vi "1_SimpleDemo_MHHisto.vi"() -> ()   [LabVIEW 2017]
uses:
  _lib/PQ/MultiHarp/MH_RefSource.ctl
  _lib/PQ/MultiHarp/MH_MeasMode.ctl
  _lib/PQ/MultiHarp/mhlib_x86_x64_UIThread.llb/MH_DllPath_global.vi
  <vilib>/Utility/error.llb/Error Cluster From Error Code.vi
  _lib/PQ/MultiHarp/MH_LibVersion_global.vi
  <vilib>/ErrorRing/Error Ring.xnode
panel:
  in  "Binning":i32(ring) caption="Resolution [ps]" items=["80", "160", "320", "640", "1280", "2560", "5120", "10240", "20480", "40960", "81920", "163840", "327680", "655360", "1310720", "2621440", "5242880", "10485760", "20971520", "41943040", "83886080", "167772160", "335544320"]
  in  "HistoLength":i32(ring)=6 caption="Histo Length" items=["1024", "2048", "4096", "8192", "16384", "32768", "65536"]
  in  "Acqu.Time":i32=10000 caption="Acqu.Time [ms]" min=1 max=360000 step=1
  in  "GlobalOffset":i32 caption="GlobalOffset [ns]" min=0 max=100000000 step=1
  in  "OverflowLevel":u32=65535 min=1 step=1
  in  "StopOnOverflow":bool=TRUE
  in  "Trg.Edge":i32(ring) items=["falling", "rising"]
  in  "Trg.Level":i32=-50 caption="Trg.Level [mV]" min=-1200 max=1200 step=1
  in  "Offset":i32 caption="Offset [ps]" min=-99999 max=99999 step=1
  in  "Enable":bool=TRUE
  in  "SyncTrg.Edge":i32(ring) items=["falling", "rising"]
  in  "SyncTrg.Level":i32=-50 caption="SyncTrg.Level [mV]" min=-1200 max=1200 step=1
  in  "SyncOffset":i32 caption="SyncOffset [ps]" min=-99999 max=99999 step=1
  in  "SyncDivider":i32(ring)=8 items=["1"=1, "2"=2, "4"=4, "8"=8, "16"=16]
  out "HistoGraph":T1(graph)={0.0, "Resolution"=0.08, "Histogram"=[]}
  out "CountRates":i32[](array[numeric]) caption="Count Rates [cps]"
  out "SyncRate":i32 caption="Sync Rate [cps]"
  in  "stop":bool
  out "error out":errorcluster
  # "Acquisition"
  # "All Channels"
  # "Sync"
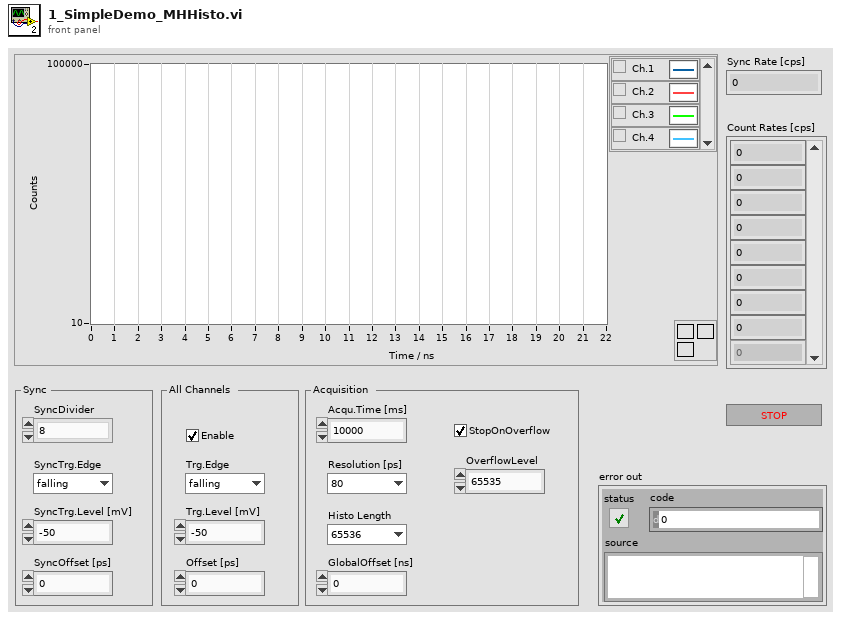
[diagram p1: front panel]
types:
  T1 = cluster{dbl, "Resolution":dbl, "Histogram":u32[][]}
  T2 = typedef "MH_MeasMode.ctl" = i32
  T3 = typedef "MH_RefSource.ctl" = enum16{"INTERNAL", "EXTERNAL_10MHZ", "WR_MASTER_GENERIC", "WR_SLAVE_GENERIC", "WR_GRANDM_GENERIC", "EXTN_GPS_PPS", "EXTN_GPS_PPS_UART", "WR_MASTER_MHARP", "WR_SLAVE_MHARP", "WR_GRANDM_MHARP"}
  T4 = typedef "MH_InitInfo.ctl" = cluster{"Library Version":string, "Serial No.":string, "Model":string, "Partnum":string, "Version":string, "features":i32, "nchannels":i32, "Base Resolution":dbl, "Bin Steps":i32}
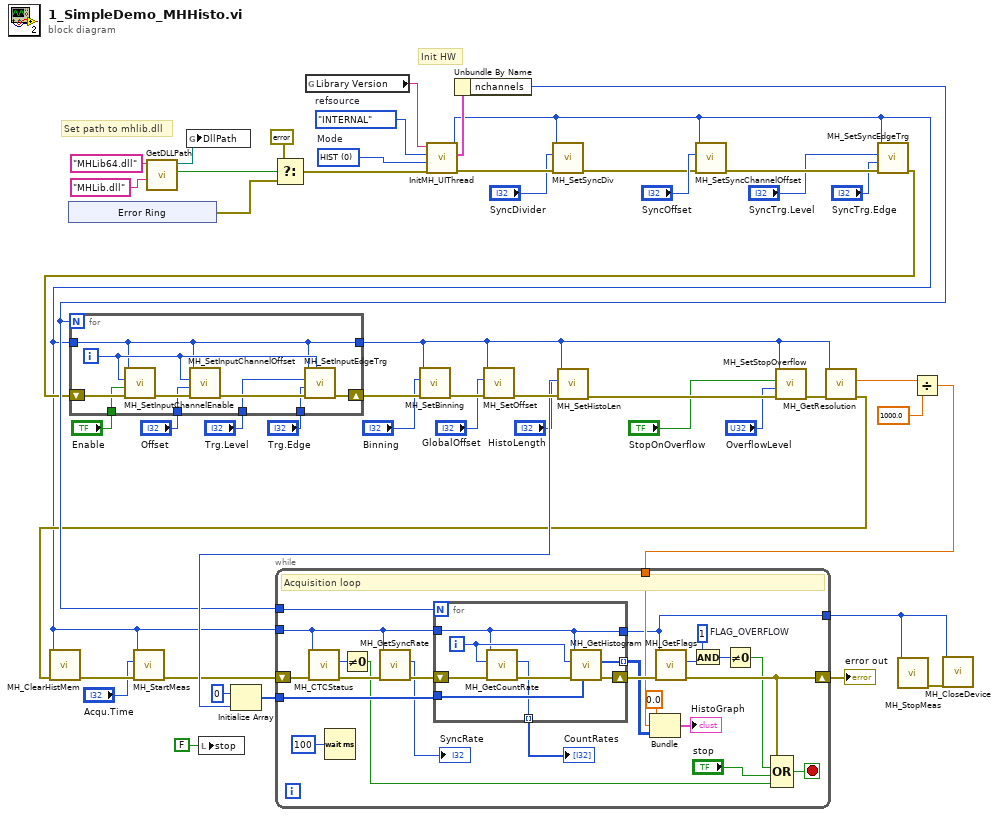
[diagram p0: block diagram]
diagram:
  w1 = T2 0 items=["HIST"=0, "T2"=2, "T3"=3]  # Mode
  w50 = MH_RefSource."INTERNAL"  # refsource
  # "Init HW"
  # "Set path to mhlib.dll"
  n1 = xnode "Error Ring"() -> ("error out"=w49:errorcluster)
  n2 = call "GetDLLPath.vi"("DllName_32bit"="MHLib.dll" ("name or relative path"), "DllName_64bit"="MHLib64.dll" ("name or relative path")) -> ("file exists?"=w47:bool, "DLLPath"=w46:path)  [unwired: 8 in]
  n3 = global write "MH_DllPath_global.vi" "DllPath"(w46) -> ()
  n4 = local write "stop"(FALSE ("stop")) -> ()
  n5 = Select(t=errorcluster {"status"=FALSE, "code"=0, "source"=""} ("error IO"), s=w47, f=w49) -> (s? t:f=w43:errorcluster)
  n6 = global read "MH_LibVersion_global.vi" "Library Version"() -> (w4:string)
  n7 = call "InitMH_UIThread.vi"("error in (no error)"=w43, "Mode"=w1, "refsource"=w50, "Library Version"=w4) -> ("error out"=w37:errorcluster, "Init Info"=w39:T4, "DevIdx"=w10:i32)  [unwired: 5 in]
  n8 = Unbundle By Name(w39) -> ("nchannels"=w19:i32)
  n9 = call "MH_SetSyncDiv.vi"("error in (no error)"=w37, "SyncDivider"="SyncDivider", "devidx"=w10) -> ("error out"=w36:errorcluster)  [unwired: 7 in, 1 out]
  n10 = call "MH_SetSyncChannelOffset.vi"("error in (no error)"=w36, "Offset"="SyncOffset", "devidx"=w10) -> ("error out"=w41:errorcluster)  [unwired: 7 in, 1 out]
  n11 = call "MH_SetSyncEdgeTrg.vi"("error in (no error)"=w41, "edge"="SyncTrg.Edge", "level"="SyncTrg.Level", "devidx"=w10) -> ("error out"=w18:errorcluster)  [unwired: 6 in, 1 out]
  n12 = for {
    N: w19 -> [_]
    shift-right: [w57] -> w38
    shift-left: w18 -> [w60]
    tunnel: w10 -> [w55]
    tunnel: [w55] -> w13
    tunnel: "Enable" -> [w54]
    tunnel: "Offset" -> [w53]
    tunnel: "Trg.Edge" -> [w52]
    tunnel: "Trg.Level" -> [w51]
    i -> [w56]
    n13 = call "MH_SetInputChannelEnable.vi"("error in (no error)"=w60, "enable"=w54, "channel"=w56, "devidx"=w55) -> ("error out"=w59:errorcluster)  [unwired: 6 in, 1 out]
    n14 = call "MH_SetInputChannelOffset.vi"("error in (no error)"=w59, "Offset"=w53, "channel"=w56, "devidx"=w55) -> ("error out"=w58:errorcluster)  [unwired: 6 in, 1 out]
    n15 = call "MH_SetInputEdgeTrg.vi"("channel"=w56, "error in (no error)"=w58, "edge"=w52, "level"=w51, "devidx"=w55) -> ("error out"=w57:errorcluster)  [unwired: 5 in, 1 out]
  }
  n16 = call "MH_SetBinning.vi"("error in (no error)"=w38, "Binning"="Binning", "devidx"=w13) -> ("error out"=w34:errorcluster)  [unwired: 7 in, 1 out]
  n17 = call "MH_SetOffset.vi"("error in (no error)"=w34, "Offset"="GlobalOffset", "devidx"=w13) -> ("error out"=w32:errorcluster)  [unwired: 7 in, 1 out]
  n18 = call "MH_SetHistoLen.vi"("error in (no error)"=w32, "lencode"="HistoLength", "devidx"=w13) -> ("error out"=w31:errorcluster, "actuallen"=w24:i32)  [unwired: 6 in, 1 out]
  n19 = Initialize Array(u32 0, w24) -> (w23:u32[])
  n20 = call "MH_SetStopOverflow.vi"("error in (no error)"=w31, "stopcount"="OverflowLevel", "StopOnOverflow"="StopOnOverflow", "devidx"=w13) -> ("error out"=w14:errorcluster)  [unwired: 6 in, 1 out]
  n21 = call "MH_GetResolution.vi"("error in (no error)"=w14, "devidx"=w13) -> ("error out"=w11:errorcluster, "resolution"=w12:dbl)  [unwired: 7 in, 1 out]
  n22 = call "MH_ClearHistMem.vi"("error in (no error)"=w11, "devidx"=w10) -> ("error out"=w28:errorcluster)  [unwired: 8 in, 1 out]
  n23 = call "MH_StartMeas.vi"("error in (no error)"=w28, "tacq"="Acqu.Time", "devidx"=w10) -> ("error out"=w9:errorcluster)  [unwired: 7 in, 1 out]
  n24 = Divide(x=w12, y=1000.0) -> (x/y=w20:dbl)
  n25 = while {
    shift-right: [w72] -> w26
    shift-left: w9 -> [w83]
    tunnel: w10 -> [w79]
    tunnel: w19 -> [w82]
    tunnel: w23 -> [w74]
    tunnel: w20 -> [w66]
    tunnel: [w61] -> w3
    stop <- w73 stop-if-true
    w77 = 1  # FLAG_OVERFLOW
    # "Acquisition loop"
    n26 = call "MH_CTCStatus.vi"("error in (no error)"=w83, "devidx"=w79) -> ("error out"=w81:errorcluster, "ctcstatus"=w84:i32)  [unwired: 7 in, 1 out]
    n27 = Wait (ms)(milliseconds to wait=u32 100) -> ()  [unwired: 1 out]
    n28 = Not Equal To 0?(x=w84) -> (x != 0?=w63:bool)
    n29 = call "MH_GetSyncRate.vi"("error in (no error)"=w81, "devidx"=w79) -> ("error out"=w80:errorcluster, "syncrate"=→"SyncRate":i32)  [unwired: 7 in, 1 out]
    n30 = for {
      N: w82 -> [_]
      shift-right: [w92] -> w78
      shift-left: w80 -> [w91]
      tunnel: w79 -> [w88]
      tunnel: [w88] -> w61
      tunnel: w74 -> [w87]
      tunnel: [w86] -> w69 mode=indexing
      tunnel: [w85] -> w68 mode=indexing
      i -> [w89]
      n31 = call "MH_GetCountRate.vi"("error in (no error)"=w91, "Channel"=w89, "devidx"=w88) -> ("error out"=w90:errorcluster, "rate"=w86:i32)  [unwired: 6 in, 1 out]
      n32 = call "MH_GetHistogram.vi"("Chcount"=w87, "error in (no error)"=w90, "channel"=w89, "devidx"=w88) -> ("error out"=w92:errorcluster, "Histogram"=w85:u32[])  [unwired: 5 in, 1 out]
    }
    "CountRates" <- w69
    n33 = Bundle(0.0, w66, "Histogram"=w68) -> (→"HistoGraph":cluster{dbl, dbl, "Histogram":u32[][]})  [unwired: 1 in]
    n34 = call "MH_GetFlags.vi"("error in (no error)"=w78, "devidx"=w61) -> ("error out"=w72:errorcluster, "flags"=w75:i32)  [unwired: 7 in, 1 out]
    n35 = And(x=w77, y=w75) -> (x .and. y?=w76:i32)
    n36 = Not Equal To 0?(x=w76) -> (x != 0?=w71:bool)
    n37 = Compound Arithmetic op=OR(w72, w71, "stop", w63) -> (w73:bool)
  }
  "error out" <- w26
  n38 = call "MH_StopMeas.vi"("devidx"=w3) -> ("error out"=w2:errorcluster)  [unwired: 9 in, 1 out]
  n39 = call "MH_CloseDevice.vi"("error in (no error)"=w2, "devidx"=w3) -> ()  [unwired: 8 in, 2 out]
